vi "电导率_所有参数读取.vi"(8 "error in (no error)":errorcluster caption="错误输入（无错误）", 11 "MB session in":refnum<class "MB_Master.lvclass">) -> (0 "error out":errorcluster caption="错误输出", 2 "输出值":T1 {"电极型号标志" items=["NULL", "pH", "Cond", "DO", "Turb"]; "电极状态标志" items=["OK"]}, 3 "MB session out":refnum<class "MB_Master.lvclass">)   [LabVIEW 2016, in "斯坦道多参数.lvlib"]
uses:
  <vilib>/Plasmionique/MB Master/MB_Master/MB_Master.lvclass
  <vilib>/Plasmionique/MB Master/MB Master.lvlib
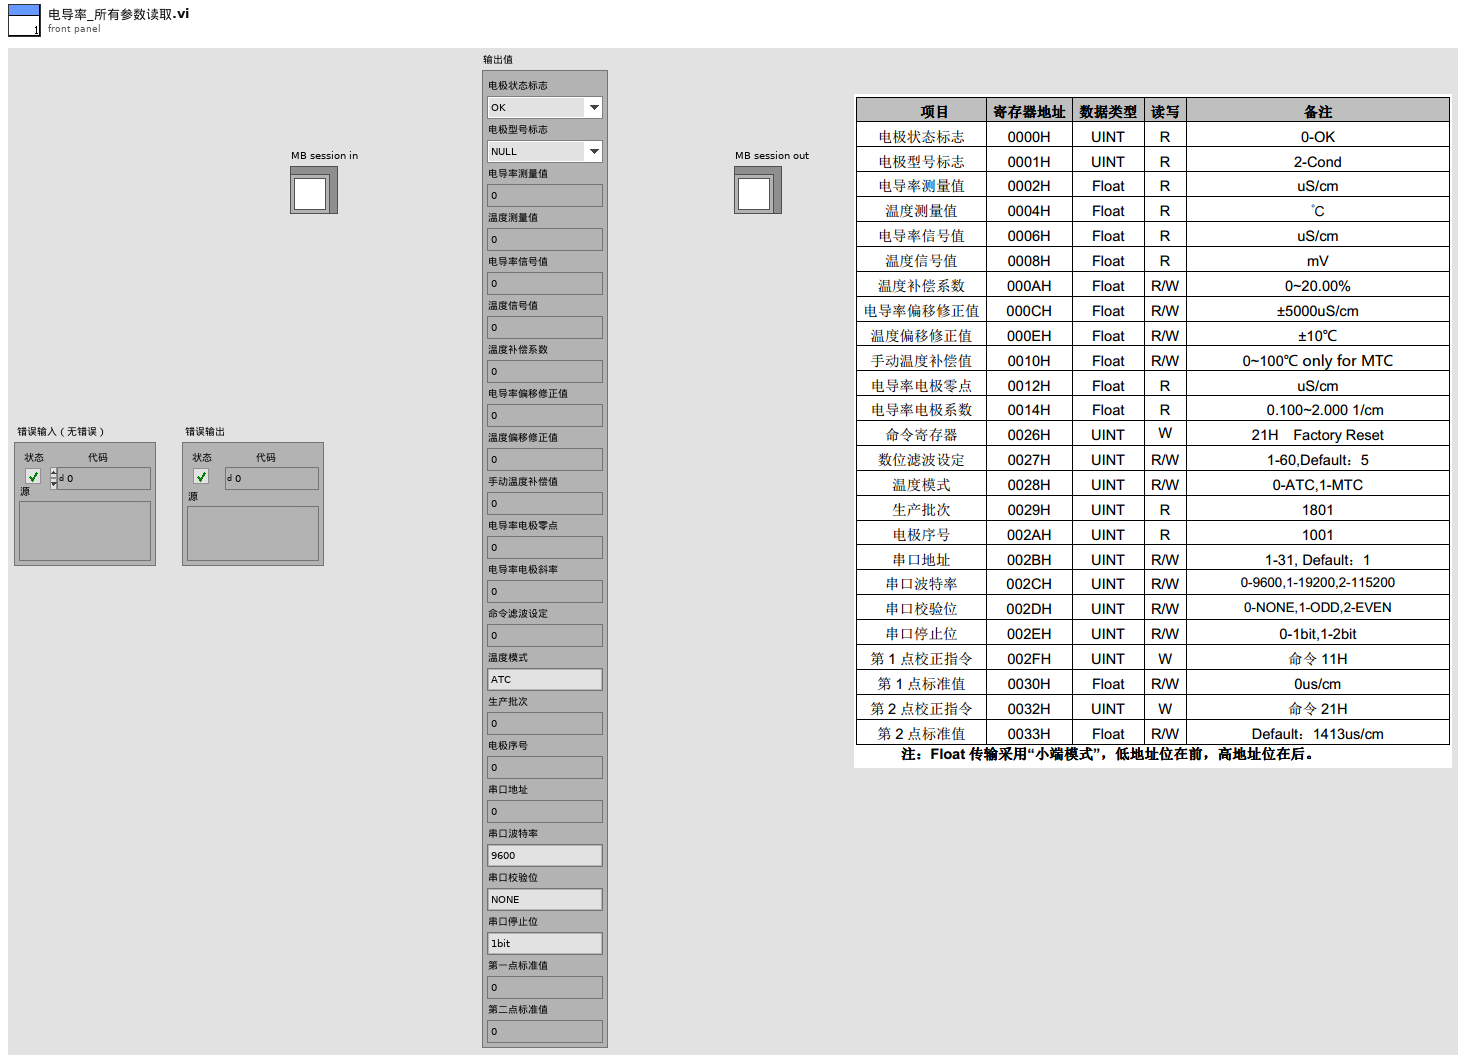
[diagram p1: front panel]
types:
  T1 = cluster{"电极状态标志":u16, "电极型号标志":u16, "电导率测量值":sgl, "温度测量值":sgl, "电导率信号值":sgl, "温度信号值":sgl, "温度补偿系数":sgl, "电导率偏移修正值":sgl, "温度偏移修正值":sgl, "手动温度补偿值":sgl, "电导率电极零点":sgl, "电导率电极斜率":sgl, "命令滤波设定":u16, "温度模式":enum16{"ATC", "MTC"}, "生产批次":u16, "电极序号":u16, "串口地址":u16, "串口波特率":enum16{"9600", "19200", "115200"}, "串口校验位":enum16{"NONE", "ODD", "EVEN"}, "串口停止位":enum16{"1bit", "2bit"}, "第一点标准值":sgl, "第二点标准值":sgl}
  T2 = cluster{u16, u16, "数值":sgl, "数值":sgl, "数值":sgl, "数值":sgl, "数值":sgl, "数值":sgl, "数值":sgl, "数值":sgl, "数值":sgl, "数值":sgl, u16, u16, u16, u16, u16, u16, u16, u16, "数值":sgl, "数值":sgl}
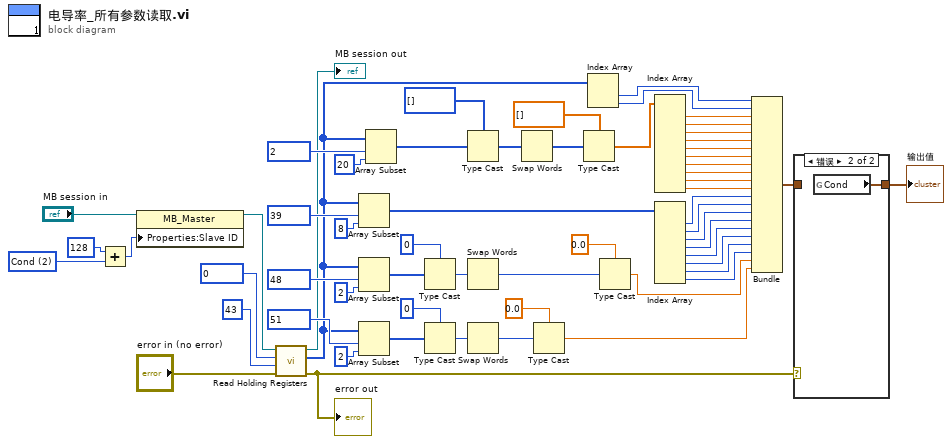
[diagram p0: block diagram]
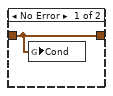
[diagram p2: hidden frame]
diagram:
  w60 = u16 2 items=["NULL", "pH", "Cond", "DO", "Turb"] ("数值")
  n1 = Add(x=u16 128, y=w60) -> (x+y=w59:u16)
  n2 = property class="MB_Master"(reference="MB session in", "Properties:Slave ID"=w59) -> (reference out=w13:refnum<class "MB_Master.lvclass">)  [unwired: 1 in, 1 out]
  n3 = call <vilib>:"Read Holding Registers.vi"("error in (no error)"="error in (no error)", "quantity"=u16 43, "starting address"=u16 0, "MB session in"=w13) -> ("error out"=w6:errorcluster, "Registers"=w27:u16[], "MB session out"=→"MB session out":refnum<class "MB_Master.lvclass">)  [unwired: 5 in]
  "error out" <- w6
  n4 = Array Subset(array=w27, index=u16 39 ("starting address"), length=8 ("长度")) -> (w40:u16[])
  n5 = Array Subset(array=w27, index=u16 48 ("starting address"), length=2 ("长度")) -> (w22:u16[])
  n6 = Array Subset(array=w27, index=u16 51 ("starting address"), length=2 ("长度")) -> (w17:u16[])
  n7 = Array Subset(array=w27, index=u16 2 ("starting address"), length=20 ("长度")) -> (w48:u16[])
  n8 = Type Cast(type=u32 0 ("数值"), x=w22) -> (*(type *) &x=w25:u32)
  n9 = Type Cast(type=u32 0 ("数值"), x=w17) -> (*(type *) &x=w19:u32)
  n10 = Type Cast(type=u32[] [] ("数组 2"), x=w48) -> (*(type *) &x=w50:u32[])
  n11 = Swap Words(1:w25) -> (0:w26:u32)
  n12 = Swap Words(1:w19) -> (0:w18:u32)
  n13 = Swap Words(1:w50) -> (0:w52:u32[])
  n14 = Type Cast(type=sgl 0.0 ("数值"), x=w18) -> (*(type *) &x=w15:sgl)
  n15 = Type Cast(type=sgl[] [] ("数组 2"), x=w52) -> (*(type *) &x=w47:sgl[])
  n16 = Index Array(array=w27) -> (element #1=w55:u16, element #2=w54:u16)  [unwired: 2 in]
  n17 = Type Cast(type=sgl 0.0 ("数值"), x=w26) -> (*(type *) &x=w16:sgl)
  n18 = Index Array(array=w47) -> (element #1=w2:sgl, element #2=w46:sgl, element #3=w45:sgl, element #4=w44:sgl, element #5=w12:sgl, element #6=w11:sgl, element #7=w10:sgl, element #8=w9:sgl, element #9=w8:sgl, element #10=w7:sgl)  [unwired: 10 in]
  n19 = Index Array(array=w40) -> (element #1=w39:u16, element #2=w38:u16, element #3=w37:u16, element #4=w36:u16, element #5=w35:u16, element #6=w34:u16, element #7=w33:u16, element #8=w32:u16)  [unwired: 8 in]
  n20 = Bundle(w55, w54, "数值"=w2, "数值"=w46, "数值"=w45, "数值"=w44, "数值"=w12, "数值"=w11, "数值"=w10, "数值"=w9, "数值"=w8, "数值"=w7, w39, w38, w37, w36, w35, w34, w33, w32, "数值"=w16, "数值"=w15) -> (w5:T2)  [unwired: 1 in]
  n21 = case shown="错误" w6 {
    tunnel: w5 -> [w61 _]
    tunnel: [w61 w62] -> w1
    frame No Error {
      n22 = global write "国弘过程全局变量.vi" "Cond"(w61) -> ()
    }
    frame Error {
      n23 = global read "国弘过程全局变量.vi" "Cond"() -> (w62:T1)
    }
  }
  "输出值" <- w1
